vi "X stage safety.vi"(7 "new position":dbl format="%#_13g", 8 "Error In":errorcluster, 10 "Table Stages":T1={"X Stage"={"Position"=0.0, "Is.Enabled?"=FALSE, "Is.Connected?"=FALSE, "Device SN"="45876539", "AccelerationMaximum"=0.0, "VelocityMaximum"=0.0, "Acceleration"=0.0, "Velocity"=0.0, "waitTimeout (ms)"=0, "Model"=enum."None", "Is.Homed?"=FALSE, "MOVE"=FALSE}, "Y Stage"={"Position"=0.0, "Is.Enabled?"=FALSE, "Is.Connected?"=FALSE, "Device SN"="45876539", "AccelerationMaximum"=0.0, "VelocityMaximum"=0.0, "Acceleration"=0.0, "Velocity"=0.0, "waitTimeout (ms)"=0, "Model"=enum."None", "Is.Homed?"=FALSE, "MOVE"=FALSE}, "Z Stage"={"Position"=0.0, "Is.Enabled?"=FALSE, "Is.Connected?"=FALSE, "Device SN"="45876539", "AccelerationMaximum"=0.0, "VelocityMaximum"=0.0, "Acceleration"=0.0, "Velocity"=0.0, "waitTimeout (ms)"=0, "Model"=enum."None", "Is.Homed?"=FALSE, "MOVE"=FALSE}, "Attenuator"={"Position"=0.0, "Is.Enabled?"=FALSE, "Is.Connected?"=FALSE, "Device SN"="45876539", "AccelerationMaximum"=0.0, "VelocityMaximum"=0.0, "Acceleration"=0.0, "Velocity"=0.0, "waitTimeout (ms)"=0, "Model"=enum."None", "Is.Homed?"=FALSE, "MOVE"=FALSE}}) -> (0 "Error Out":errorcluster, 1 "crash?":bool)   [LabVIEW 2018]
uses:
  Controls/Translation Stage Parameters.ctl
  Hardware Mfg/Thorlabs Translation Stages/Controls/Translation Stage Cluster.ctl
  Controls/Translation Stage Types.ctl
  Controls/Set Get Controls.ctl
  Hardware Mfg/Thorlabs Translation Stages/Controls/Motion Translation Module Control2.ctl
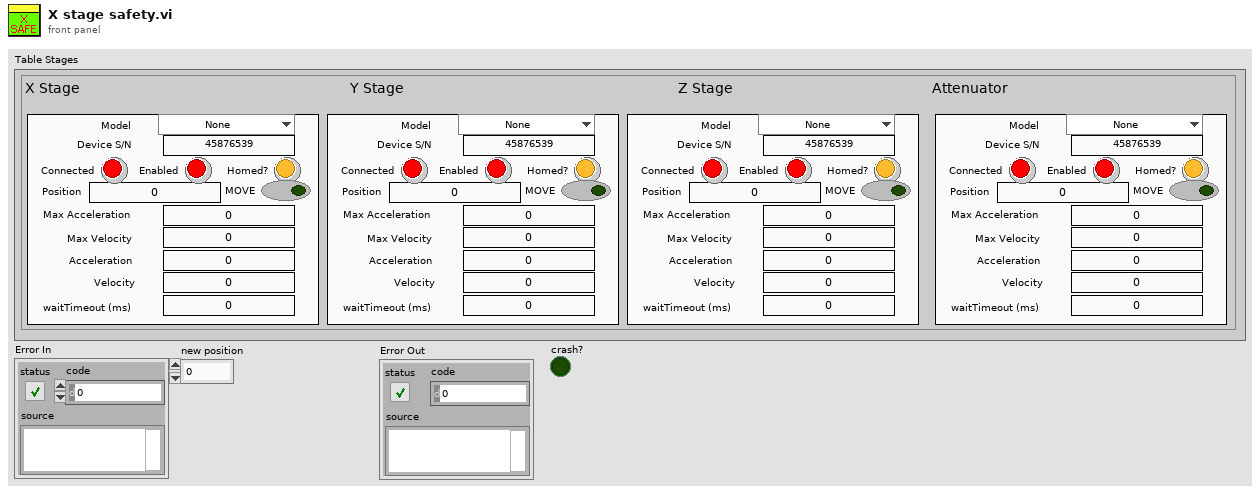
[diagram p1: front panel]
types:
  T1 = typedef "Translation Stage Parameters.ctl" = cluster{"X Stage":T2, "Y Stage":T2, "Z Stage":T2, "Attenuator":T2}
  T2 = typedef "Translation Stage Cluster.ctl" = cluster{"Position":dbl, "Is.Enabled?":bool, "Is.Connected?":bool, "Device SN":string, "AccelerationMaximum":dbl, "VelocityMaximum":dbl, "Acceleration":dbl, "Velocity":dbl, "waitTimeout (ms)":i32, "Model":T3, "Is.Homed?":bool, "MOVE":bool}
  T3 = typedef "Translation Stage Types.ctl" = enum16{"None", "Thorlabs LTS", "Thorlabs MLJ"}
  T4 = typedef "Motion Translation Module Control2.ctl" = enum16{"Init", "Home", "Status", "Velocity/Accel", "Position", "Jog", "Stop", "Uninit", "Enable", "Disable"}
  T5 = typedef "Set Get Controls.ctl" = enum16{"Set", "Get"}
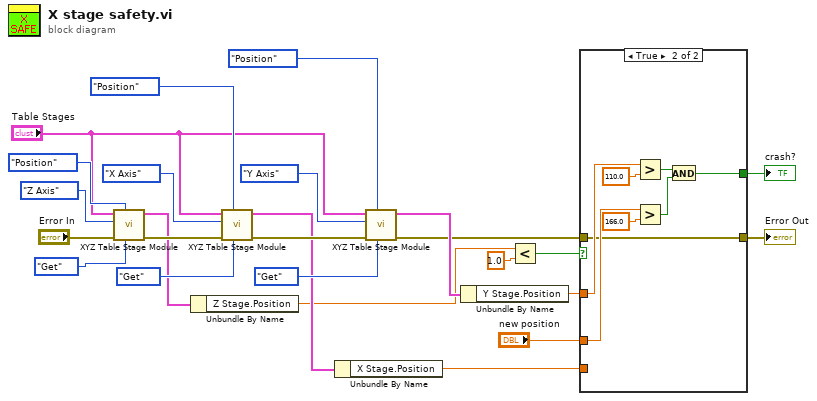
[diagram p0: block diagram]
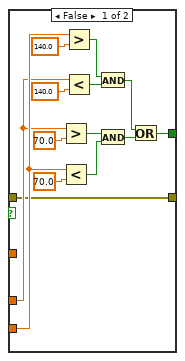
[diagram p2: hidden frame]
diagram:
  n1 = call "XYZ Table Stage Module.vi"("Set/Get"=Set_Get_Controls."Get", "Action"=Motion_Translation_Module_Control2."Position", "Error In"="Error In", "Axis"=enum16{"X Axis", "Y Axis", "Z Axis"}."Z Axis", "Table Stages"="Table Stages") -> ("Error Out"=w18:errorcluster, "Table Stages [out]"=w13:T1)  [unwired: 5 in]
  n2 = Unbundle By Name(w13) -> ("Z Stage.Position"=w10:dbl)
  n3 = call "XYZ Table Stage Module.vi"("Set/Get"=Set_Get_Controls."Get", "Action"=Motion_Translation_Module_Control2."Position", "Error In"=w18, "Axis"=enum16{"X Axis", "Y Axis", "Z Axis"}."X Axis", "Table Stages"="Table Stages") -> ("Error Out"=w14:errorcluster, "Table Stages [out]"=w11:T1)  [unwired: 5 in]
  n4 = Unbundle By Name(w11) -> ("X Stage.Position"=w4:dbl)
  n5 = call "XYZ Table Stage Module.vi"("Set/Get"=Set_Get_Controls."Get", "Action"=Motion_Translation_Module_Control2."Position", "Error In"=w14, "Axis"=enum16{"X Axis", "Y Axis", "Z Axis"}."Y Axis", "Table Stages"="Table Stages") -> ("Error Out"=w2:errorcluster, "Table Stages [out]"=w12:T1)  [unwired: 5 in]
  n6 = Unbundle By Name(w12) -> ("Y Stage.Position"=w6:dbl)
  n7 = Less?(x=w10, y=1.0) -> (x < y?=w8:bool)
  n8 = case shown="True" w8 {
    tunnel: "new position" -> [w32 w47]
    tunnel: w6 -> [_ w45]
    tunnel: [w27 w41] -> w5
    tunnel: w4 -> [w33 _]
    tunnel: w2 -> [w26 w40]
    tunnel: [w26 w40] -> w1
    frame False {
      n9 = Greater?(x=w32, y=70.0) -> (0:w31:bool)
      n10 = Less?(x=w33, y=70.0) -> (x < y?=w30:bool)
      n11 = Greater?(x=w33, y=140.0) -> (0:w37:bool)
      n12 = Less?(x=w32, y=140.0) -> (x < y?=w36:bool)
      n13 = And(x=w37, y=w36) -> (x .and. y?=w29:bool)
      n14 = And(x=w31, y=w30) -> (x .and. y?=w28:bool)
      n15 = Or(x=w29, y=w28) -> (x .or. y?=w27:bool)
    }
    frame True {
      n16 = Greater?(x=w45, y=110.0) -> (0:w43:bool)
      n17 = Greater?(x=w47, y=166.0) -> (0:w42:bool)
      n18 = And(x=w43, y=w42) -> (x .and. y?=w41:bool)
    }
  }
  "crash?" <- w5
  "Error Out" <- w1
